vi "finishup.vi"(8 "error in (no error)":errorcluster, 11 "AnalysisResultsViewer in":refnum<class "AnalysisResultsViewer.lvclass">) -> (0 "error out":errorcluster, 3 "AnalysisResultsViewer out":refnum<class "AnalysisResultsViewer.lvclass">)   [LabVIEW 2009, in "Views.lvlib" / "Camera.lvlib" / "AnalysisResultsViewer.lvclass"]
uses:
  AnalysisResultsViewer.lvclass
  AnalysisResultsViewer.lvclass/AnalysisResultsViewer.ctl
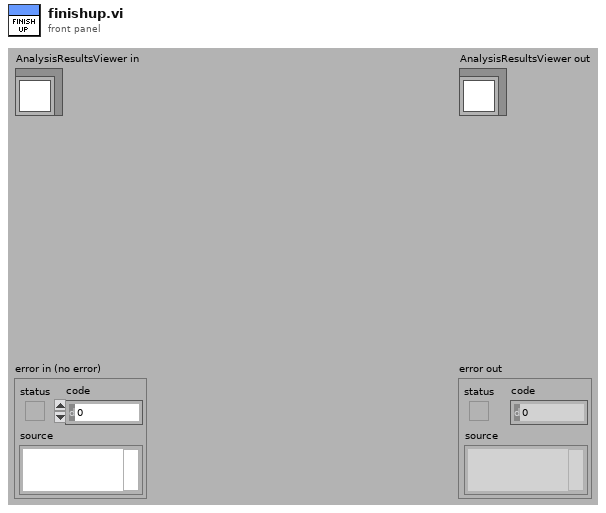
[diagram p1: front panel]
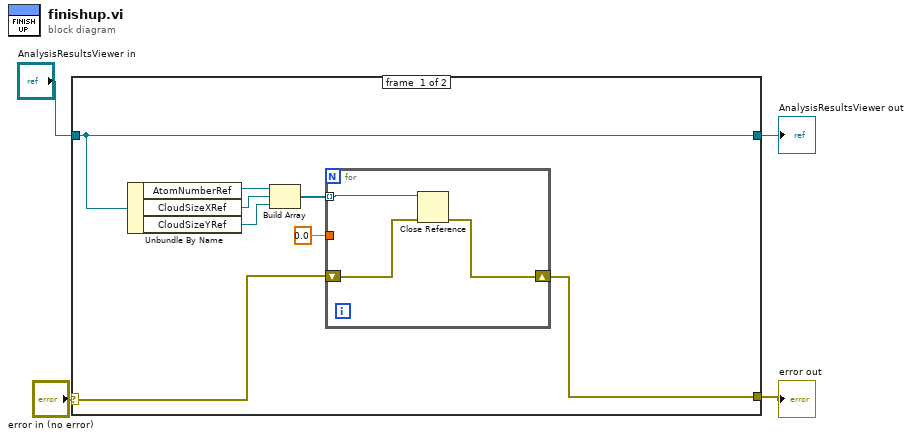
[diagram p0: block diagram]
diagram:
  n1 = case shown="No Error" "error in (no error)" {
    selector: "error in (no error)" -> [w7 w17]
    tunnel: [w6 w17] -> w3
    tunnel: [w5 w16] -> w1
    tunnel: "AnalysisResultsViewer in" -> [w5 w16]
    frame #0 {
      n2 = Unbundle By Name(w5) -> ("AtomNumberRef"=w12:refnum<vi>, "CloudSizeXRef"=w11:refnum<vi>, "CloudSizeYRef"=w10:refnum<vi>)
      n3 = Build Array(w12, w11, w10) -> (w9:refnum<vi>[])
      n4 = for {
        tunnel: w9 -> [w15] mode=indexing
        tunnel: 0.0 -> [_]
        shift-right: [w13] -> w6
        shift-left: w7 -> [w14]
        n5 = Close Reference(reference=w15, error in (no error)=w14) -> (error out=w13:errorcluster)
      }
    }
    frame #1 {
    }
  }
  "error out" <- w3
  "AnalysisResultsViewer out" <- w1
